vi "Get Next 429 Record In Reader.vi"(8 "error in (no error)":errorcluster, 11 "core reader handle in":u64) -> (0 "error out":errorcluster, 2 "record out":T1 {"type" format="%04x"; "timestamp" format="%08x"; "msgact" format="%04x"; "data" format="%08x"; "timestamph" format="%08x"}, 3 "core reader handle out":u64)   [LabVIEW 2020, in "Ballard ARINC 429 Hardware API.lvlib"]
doc: "Retrieves the next 429 record from the reader associated with <B>core reader handle in</B>. If no record is found, an error is returned.\n\nVerify the reader actually holds data by using the <B>records read</B> indicator returned by the <B>Read</B> VI."
uses:
  <instrlib>/BTICardLib/Public/Controls/429 Record.ctl
  Ballard ARINC 429 Hardware API.lvlib
  BTICardLV.dll
  <instrlib>/BTICardLib/BTICardLV.lvlib
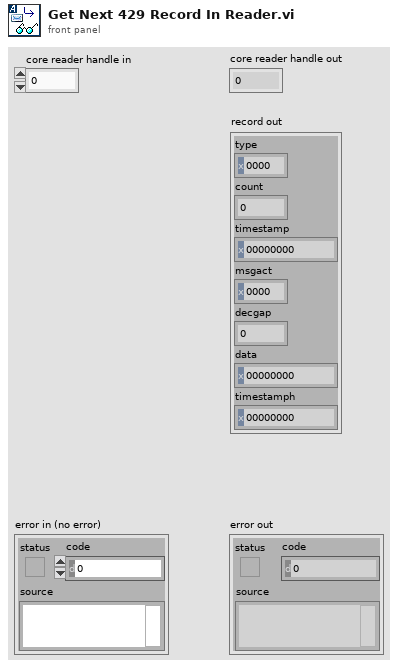
[diagram p1: front panel]
types:
  T1 = typedef "BTICardLV.lvlib/429 Record.ctl" = cluster{"type":u16, "count":u16, "timestamp":u32, "msgact":u16, "decgap":u16, "data":u32, "timestamph":u32}
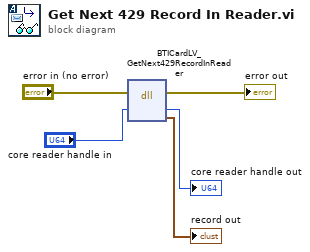
[diagram p0: block diagram]
diagram:
  n1 = dll-call lib="BTICardLV.*" fn="BTICardLV_GetNext429RecordInReader"(error in="error in (no error)", "readerhandle"="core reader handle in") -> (error out=→"error out":errorcluster, "readerhandle"=→"core reader handle out":u64, "record out"=→"record out":T1)  [unwired: 4 in, 1 out]
